vi "WPI_DriverStationGet Robot Battery Voltage.vi"(11 "error in (no error)":errorcluster) -> (8 "robot battery voltage":dbl, 15 "error out":errorcluster)   [LabVIEW 2017]
doc: "Returns the battery voltage of the robot in the robot program. You must use this VI while the Start Communication VI is running so the program knows what battery voltage to read. The battery voltage returned in this VI is the same as the one that displays in the FRC Driver Station."
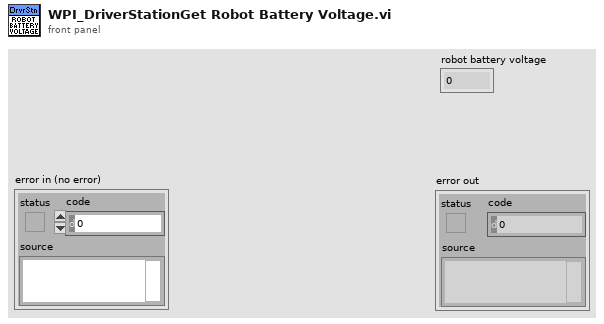
[diagram p1: front panel]
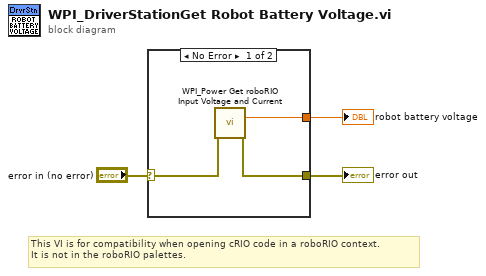
[diagram p0: block diagram]
diagram:
  # "This VI is for compatibility when opening cRIO code in a roboRIO context.\nIt is not in the roboRIO palettes."
  n1 = case shown="No Error" "error in (no error)" {
    selector: "error in (no error)" -> [w6 w7]
    tunnel: [w5 w7] -> w2
    tunnel: [w4 _] -> w1
    frame No Error {
      n2 = call <vilib>:"WPI_Power Get roboRIO Input Voltage and Current.vi"("error in"=w6) -> ("roboRIO input voltage (V)"=w4:dbl, "error out"=w5:errorcluster)  [unwired: 12 in, 1 out]
    }
    frame Error {
    }
  }
  "error out" <- w2
  "robot battery voltage" <- w1
